vi "fg.vi"() -> ()   [LabVIEW 2011]
uses:
  <vilib>/Instr/_visa.llb/VISA Configure Serial Port (Instr).vi
panel:
  in  "Wave Form":u16(ring) items=["Square", "Sawtooth", "Ramp"]
  in  "Com?":refnum<visa-resource-name>
  in  "Phase":dbl(slide) scale=-180.0..180.0
  in  "Duty Cycle (%)":dbl(knob) scale=0.0..100.0
  out "Waveform Graph":waveform(dbl)(graph)
  in  "Offset":dbl(slide) scale=-5.0..5.0
  in  "Freq.":dbl(knob) scale=1.0..400.0
  in  "Freq. Unit":u16(ring) items=["mHz", "Hz", "kHz"]
  in  "Ampl.":dbl(knob) scale=0.0..5.0
  in  "Help Button":bool
  in  "?":bool
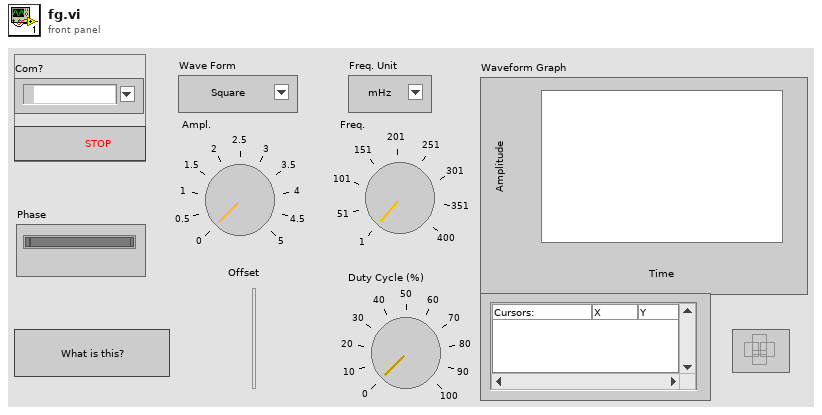
[diagram p1: front panel]
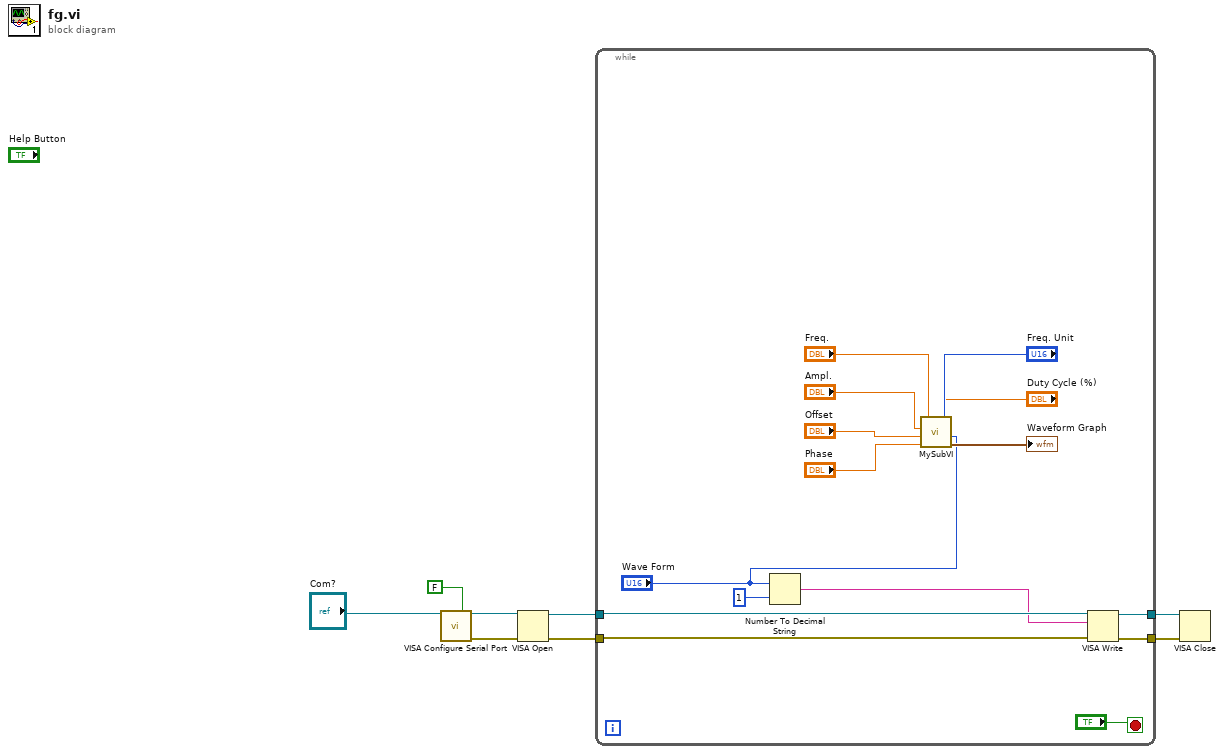
[diagram p0: block diagram]
diagram:
  n1 = call-poly "VISA Configure Serial Port"("VISA resource name"="Com?", "Enable Termination\nChar (T)"=FALSE ("Enable Termination\nChar (T)")) -> ("VISA resource name out"=w5:refnum<visa-resource-name>, "error out"=w4:errorcluster)  [unwired: 12 in]
  n2 = VISA Open(error in (no error)=w4, VISA resource name=w5) -> (VISA resource name=w2:refnum<visa-resource-name>, error out=w3:errorcluster)  [unwired: 3 in]
  n3 = while {
    tunnel: w2 -> [w12]
    tunnel: [w22] -> w8
    tunnel: w3 -> [w11]
    tunnel: [w21] -> w7
    stop <- "?" stop-if-true
    n4 = Number To Decimal String(number="Wave Form", width (-)=i16 1) -> (decimal integer string=w9:string)
    n5 = call "MySubVI.vi"("Wave Form"="Wave Form", "Freq. Unit"="Freq. Unit", "Duty Cycle (%)"="Duty Cycle (%)", "Phase"="Phase", "Offset"="Offset", "Ampl."="Ampl.", "Freq."="Freq.") -> ("Waveform Graph"=→"Waveform Graph":waveform(dbl))
    n6 = VISA Write(VISA resource name=w12, write buffer=w9, error in (no error)=w11) -> (VISA resource name out=w22:refnum<visa-resource-name>, error out=w21:errorcluster)  [unwired: 1 out]
  }
  n7 = VISA Close(VISA resource name=w8, error in (no error)=w7) -> ()  [unwired: 1 out]
